vi "Main.vi"(8 "error in (no error)":T1) -> (0 "error out":T1)   [LabVIEW 2019, in "HW Control.lvlib"]
doc: "Confgures and operates mmWave insturment.\nTakes tx data and produces rx data"
uses:
  HW Control.lvlib
  module data.ctl
  SubVIs/mmWave instrument_class/mmWave instrument.lvclass
  SubVIs/Timing_class/Timing.lvclass
  Intertarget communication/UE_slave_class/UE_slave.lvclass
  Intertarget communication/Status + response + data cluster.ctl
  <vilib>/event_ctls.llb/usereventprio.ctl
  SubVIs/mmWave instrument_class/Instrument mode.ctl
  SubVIs/Shared/CMD Configure RF.ctl
  mmw_command_lib/src_LabVIEW/mmW_commands/commands/configure_rf.ctl
  SubVIs/Shared/CMD Configure trigger.ctl
  FPGA/SubVIs/Utility/FPGA driver trigger source.ctl
  FPGA/SubVIs/Utility/FPGA driver trigger destination.ctl
  SubVIs/Low-level/TypeDefs/TX trigger config.ctl
  SubVIs/Shared/CMD SetFS.ctl
  SubVIs/Shared/CMD Enable.ctl
  SubVIs/Shared/CMD Start.ctl
  SubVIs/mmWave HW Control/HW custom error.ctl
  SubVIs/Shared/CMD Trigger burst.ctl
  SubVIs/mmWave instrument_class/BurstMode.ctl
  SubVIs/IQBurst_memo_class/IQBurst_memo.lvclass
  C:/Barkhausen mmWave radar/Development/modules/mmw_instrument/src_LabVIEW/Host/SubVIs/mmWave data_class/mmWave data.lvclass
  5bf6cc24-2521-4779-a80f-885c0f377251.vi
  6b8a8956-422c-4712-ba84-b3f6b6fa3076.vi
  cc201456-c6b0-4b1b-a6be-4740aef1e4bc.vi
  d80f0b82-403c-4990-a471-3ef8a1654657.vi
  00066108-5967-43ca-95ae-979ba40a526a.vi
  dd2405c6-cd62-4e0d-85ef-7dac0ed472a1.vi
  39e6701a-dc6a-46a4-ab36-30c5359b2d1b.vi
  9bb7bbee-87a9-4279-9159-38fc56038457.vi
  5d9b41d4-afd7-4f36-a909-48ea6e6084fe.vi
  c62d52e6-4296-4856-a5ed-4f8c0908956e.vi
  5d74ec58-d27a-4030-a0b1-2ab9eda5ed47.vi
  04c4d11f-ea94-45d4-9853-bbcd34ad9d24.vi
  03bbd1a8-d73e-4344-8b1d-11c8de24bdb2.vi
  b8e4441c-5df3-4338-bc39-36b1f38d4699.vi
  39a1d11b-c092-41e2-b849-1242f73b0438.vi
  25709526-e8ac-4911-9c95-dbb1750b9ebd.vi
  0d6dd9cf-0a41-4f7f-9007-575a6cdc04d9.vi
  c6908804-639b-480e-8665-cc71bcbfa22b.vi
  f746113e-c9c3-4718-88dd-bf493a6a5370.vi
  31d5450a-1eaa-4569-b864-abab59b6c8f0.vi
  0cf5399d-4f5c-45f4-9da5-b5ff7f003509.vi
  ffcc4e67-c424-41ae-a3a8-51a0e91b4a98.vi
  4f1527e8-8d13-40e8-9887-532582f60c4c.vi
  48a184bb-bc8e-4bef-accd-5d588c8dfd0c.vi
  281b50d0-36cb-43e3-a457-c2e31bbdf17e.vi
  6b8a8956-422c-4712-ba84-b3f6b6fa3076.vi/d0b8099d-9a67-487c-8619-7aec39155471.vi
  6b8a8956-422c-4712-ba84-b3f6b6fa3076.vi/4860adc8-6589-4533-9f85-4b2f2f37bc9c.vi
  <vilib>/Utility/High Resolution Relative Seconds.vi
  00066108-5967-43ca-95ae-979ba40a526a.vi/b21b0c59-31bf-4d41-a314-fcb12202764f.vi
  00066108-5967-43ca-95ae-979ba40a526a.vi/59aae4f2-523e-4201-a515-759cc9f383bb.vi
  9bb7bbee-87a9-4279-9159-38fc56038457.vi/ee473946-ddb2-4ec3-8c70-25ef1014e137.vi
  9bb7bbee-87a9-4279-9159-38fc56038457.vi/b9ef59a3-996d-41eb-8d73-01ad8261f39e.vi
  5d9b41d4-afd7-4f36-a909-48ea6e6084fe.vi/0198eef5-db64-4605-ab12-3a788667f18b.vi
  5d9b41d4-afd7-4f36-a909-48ea6e6084fe.vi/f3eba246-8368-4cb8-a50b-49fa0b258f31.vi
  c62d52e6-4296-4856-a5ed-4f8c0908956e.vi/b2fe2695-0bc7-407f-97cd-20d9374a95f4.vi
  c62d52e6-4296-4856-a5ed-4f8c0908956e.vi/e0a517d9-0214-4515-8cec-b207ba4c4c0e.vi
  5d74ec58-d27a-4030-a0b1-2ab9eda5ed47.vi/5a33c0d7-36a7-40b4-9b83-6d2230f6ca4f.vi
  5d74ec58-d27a-4030-a0b1-2ab9eda5ed47.vi/955e3d06-b885-4e3c-85b1-b793e0d77f43.vi
  04c4d11f-ea94-45d4-9853-bbcd34ad9d24.vi/622e0601-9f83-48d3-8254-9b6c5c72482e.vi
  04c4d11f-ea94-45d4-9853-bbcd34ad9d24.vi/4782b8fe-f5f5-46a3-8689-b75fcbd153d5.vi
  03bbd1a8-d73e-4344-8b1d-11c8de24bdb2.vi/af184250-e209-477c-8d9f-d9d37ba09fbc.vi
  03bbd1a8-d73e-4344-8b1d-11c8de24bdb2.vi/336334d0-afb7-43ed-8f90-156a38e6ec86.vi
  25709526-e8ac-4911-9c95-dbb1750b9ebd.vi/ce79f8f7-6f86-47e2-830d-b0a909de7e40.vi
  25709526-e8ac-4911-9c95-dbb1750b9ebd.vi/12f0f21d-a4f0-4ad2-89d4-91e03973e4f6.vi
  0cf5399d-4f5c-45f4-9da5-b5ff7f003509.vi/1adb11cf-635f-40ae-95a1-5f7e8c26521f.vi
  0cf5399d-4f5c-45f4-9da5-b5ff7f003509.vi/b263f872-2439-4497-9f75-8855c3fb30bf.vi
  48a184bb-bc8e-4bef-accd-5d588c8dfd0c.vi/0905219e-2f5e-4d98-acf9-48d7f689f462.vi
  48a184bb-bc8e-4bef-accd-5d588c8dfd0c.vi/bcc9b3b8-3631-40a1-b7b9-ffbaff264bb1.vi
  SubVIs/NISync_class/NISync.lvclass
  C:/Barkhausen mmWave radar/Development/modules/mmw_instrument/src_LabVIEW/Host/SubVIs/Timing_class/Timing.lvclass
  SubVIs/simSync_class/simSync.lvclass
  SubVIs/niMmWave_Transceiver_class/niMmWave_Transceiver.lvclass
  C:/Barkhausen mmWave radar/Development/modules/mmw_instrument/src_LabVIEW/Host/SubVIs/mmWave instrument_class/mmWave instrument.lvclass
  SubVIs/niMmWave_Reciever_class/niMmWave_Reciever.lvclass
  SubVIs/sim_MmW_class/sim_MmW.lvclass
  SubVIs/Shared/Comm GV.vi
  SubVIs/Shared/System GV.vi
  HW GV.vi
  <vilib>/addons/_JKI.lib/Serialization/JSON/Library/Unflatten From JSON String.vi
  Log/Log GV.vi
  SubVIs/mmWave data_class/mmWave data.lvclass
  Intertarget communication/CommandResponse communication.lvlib
  SubVIs/Shared/Shared.lvlib
  FPGA/SubVIs/Utility/FPGA Utility.lvlib
  Data Managment/DataManagment.lvlib
  SubVIs/mmWave HW Control/mmWave HW Control.lvlib
  Log/Log.lvlib
  mmw_command_lib/src_LabVIEW/mmW_commands/mmW_commands.lvlib
panel:
  out "fetch 2":dbl format="%#_6p"
  # "HW Control Main"
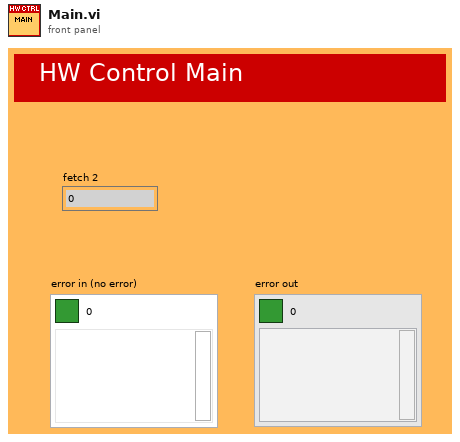
[diagram p1: front panel]
types:
  T1 = cluster{"Boolean Round":bool, "code":i32, "source":string}
  T2 = typedef "CommandResponse communication.lvlib/Status + response + data cluster.ctl" = cluster{"message":string, "response":string, "data":variant}
  T3 = typedef "HW Control.lvlib/module data.ctl" = cluster{"mmWave":refnum<class "mmWave instrument.lvclass">, "timing":refnum<class "Timing.lvclass">, "UE resp":refnum<class "UE_slave.lvclass">}
  T4 = typedef "mmWave instrument.lvclass/Instrument mode.ctl" = enum16{"RF", "IF", "BB"}
  T5 = typedef "usereventprio.ctl" = enum32{"high priority", "normal priority"}
  T6 = typedef "Shared.lvlib/CMD Configure RF.ctl" = cluster{"port":string, "fc":dbl, "gain":dbl}
  T7 = typedef "Shared.lvlib/CMD Configure trigger.ctl" = cluster{"port":string, "delay":dbl, "Trigger source":T8, "Trigger export":T9, "PXI src":i32, "PXI trigger destination":i32}
  T8 = typedef "FPGA Utility.lvlib/FPGA driver trigger source.ctl" = enum16{"Use Tclk", "PXI_Trig", "Aurora RX trig"}
  T9 = typedef "FPGA Utility.lvlib/FPGA driver trigger destination.ctl" = enum16{"None", "Source trig", "Synced trig", "Delayed sync"}
  T10 = typedef "Shared.lvlib/CMD SetFS.ctl" = cluster{"port":string, "fs":dbl}
  T11 = typedef "Shared.lvlib/CMD Enable.ctl" = cluster{"Enable":bool}
  T12 = typedef "Shared.lvlib/CMD Start.ctl" = cluster{"Bursts":string[], "Acquisition duration":dbl}
  T13 = typedef "Shared.lvlib/CMD Trigger burst.ctl" = cluster{"Burst name":string, "Burst mode":T14}
  T14 = typedef "mmWave instrument.lvclass/BurstMode.ctl" = enum16{"burst", "continuous"}
  T15 = typedef "mmW_commands.lvlib/configure_rf.ctl" = cluster{"port":enum16{"rx", "tx"}, "fc":dbl, "gain":dbl, "datatype":string}
  T16 = typedef "TX trigger config.ctl" = cluster{"delay":dbl, "trig source":T8, "PXI src":i32, "export":T9, "PXI dest":i32}
  T17 = cluster{"frequency offset (Hz)":dbl[], "response":cdb[]}
  T18 = typedef "mmWave HW Control.lvlib/HW custom error.ctl" = u16
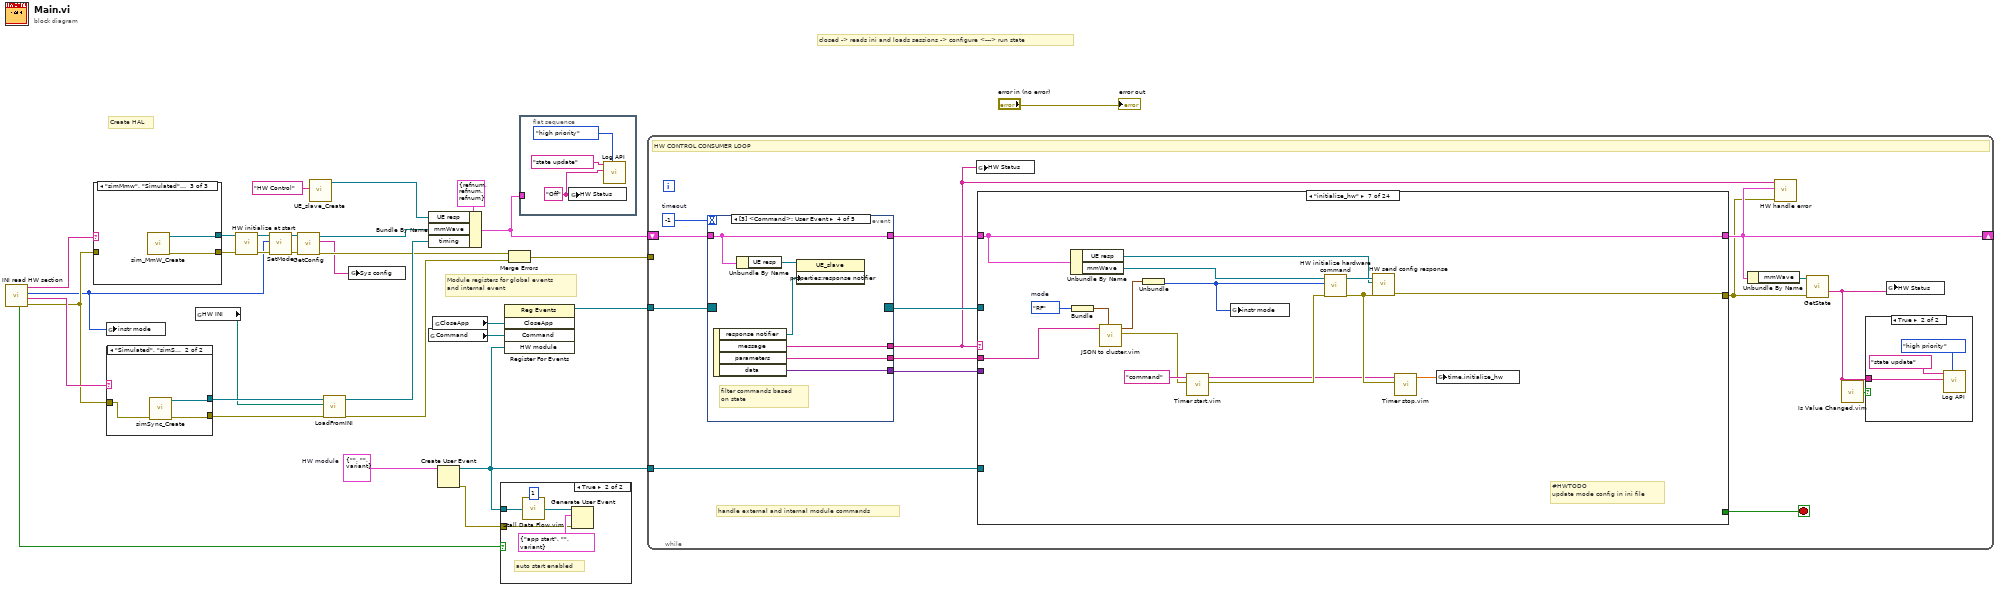
[diagram p0: block diagram]
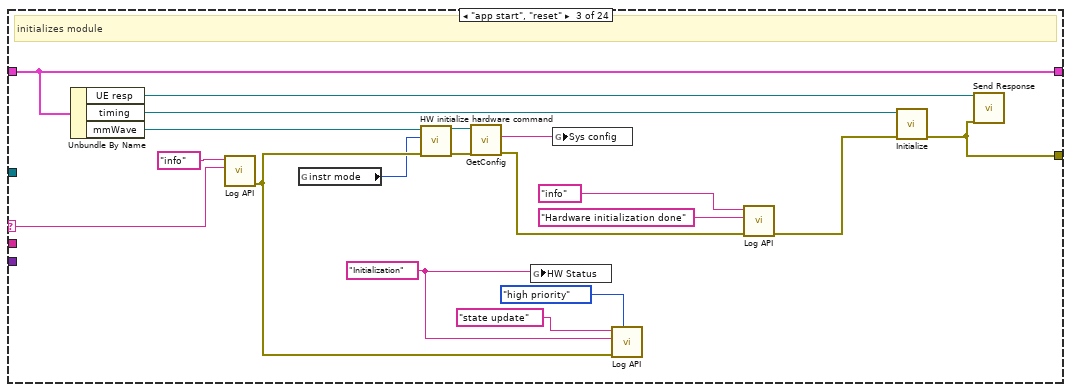
[diagram p6: hidden frame]
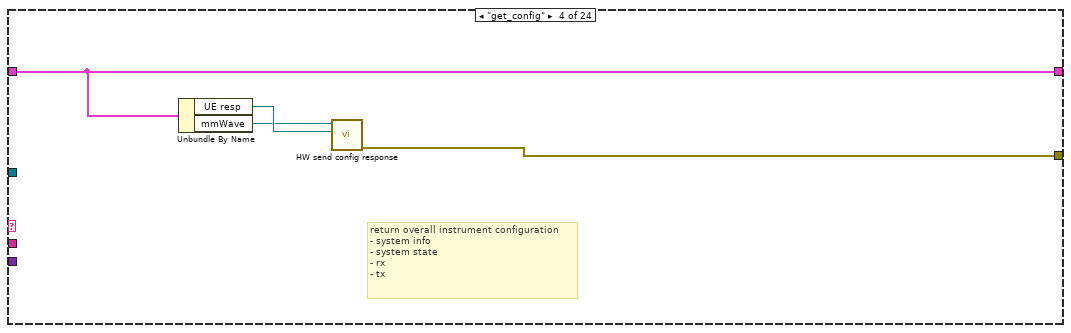
[diagram p7: hidden frame]
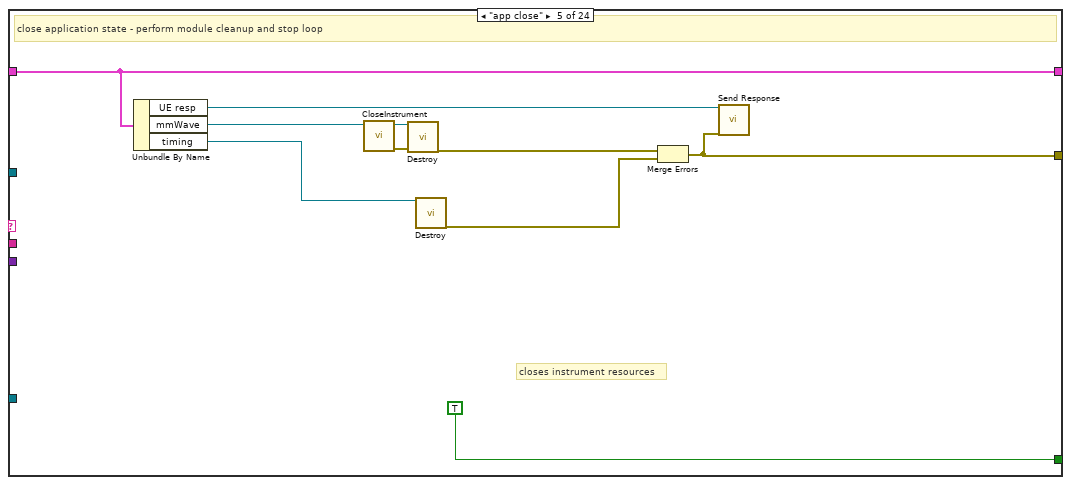
[diagram p8: hidden frame]
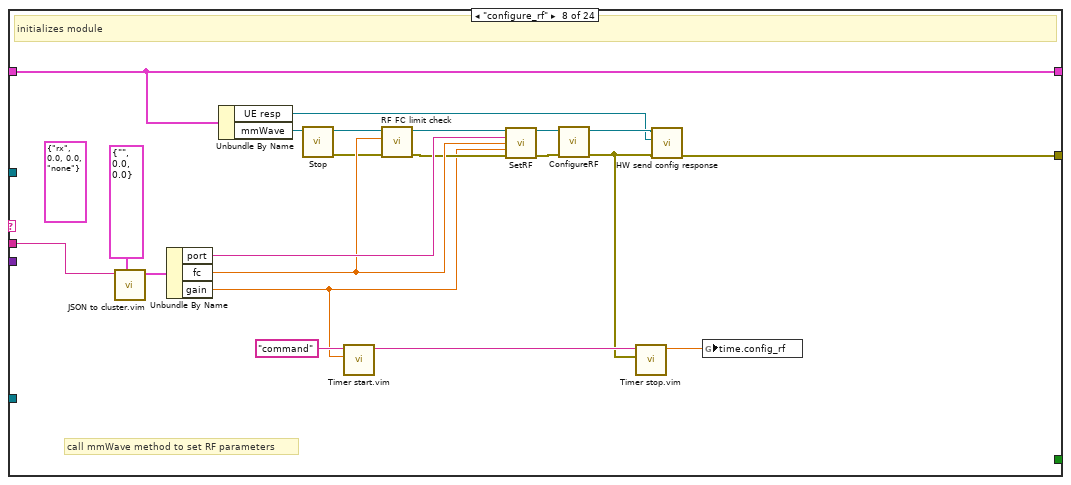
[diagram p10: hidden frame]
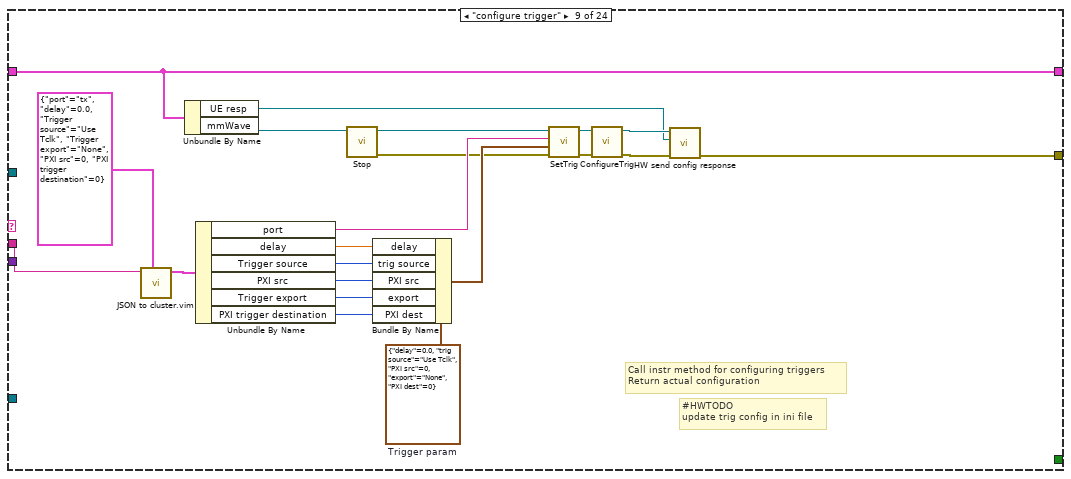
[diagram p11: hidden frame]
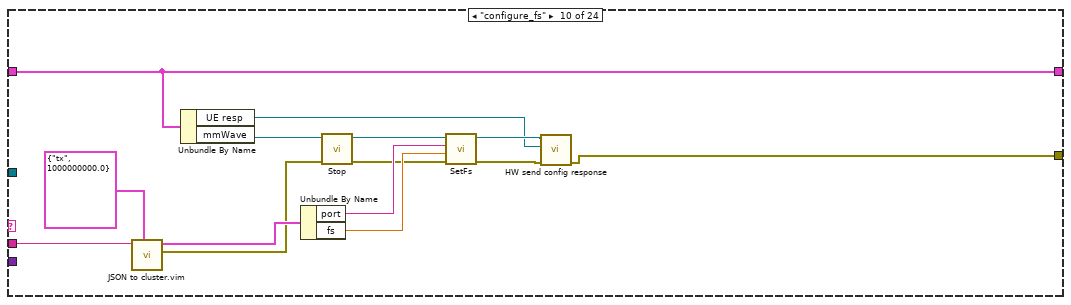
[diagram p12: hidden frame]
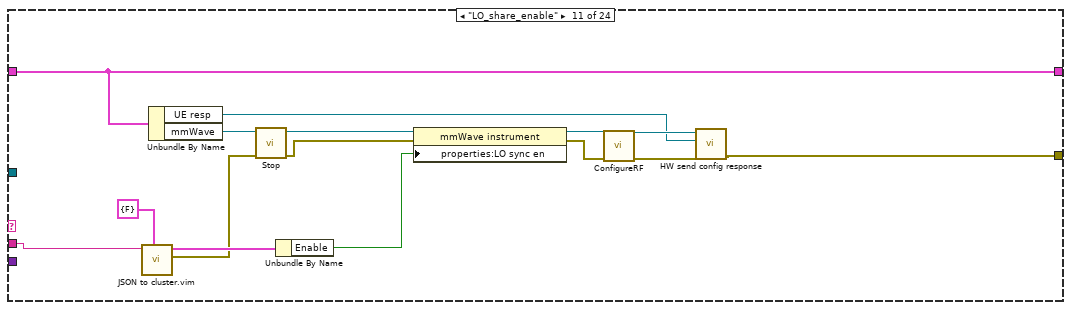
[diagram p13: hidden frame]
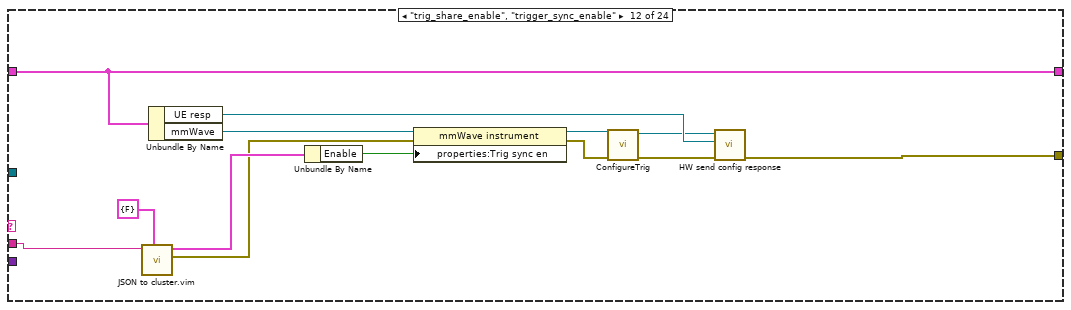
[diagram p14: hidden frame]
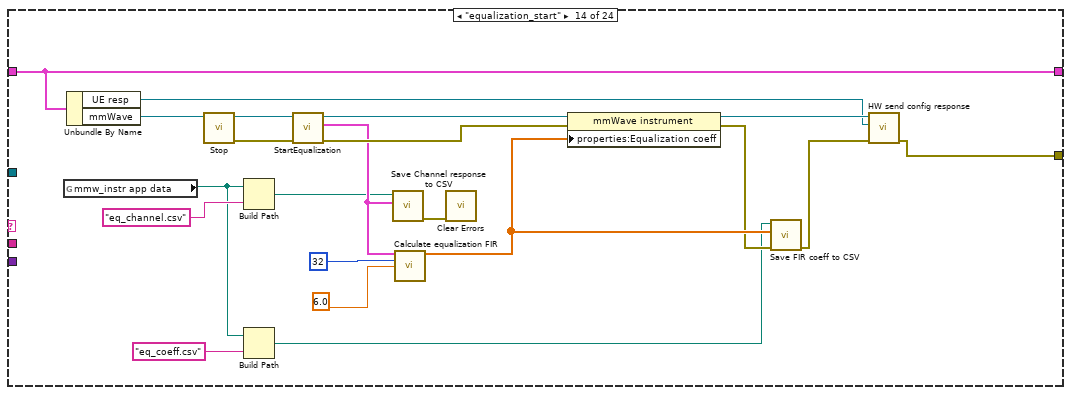
[diagram p16: hidden frame]
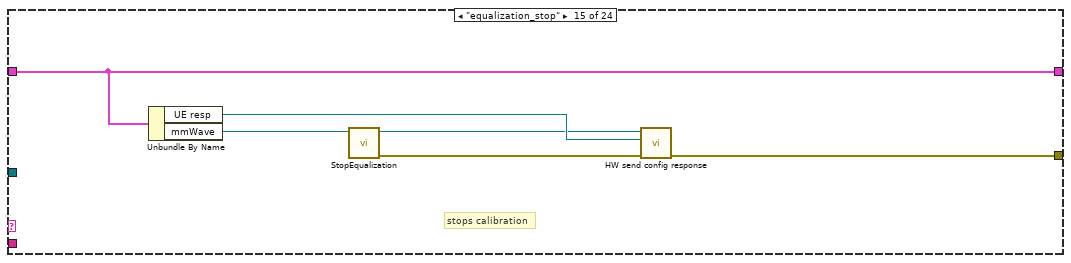
[diagram p17: hidden frame]
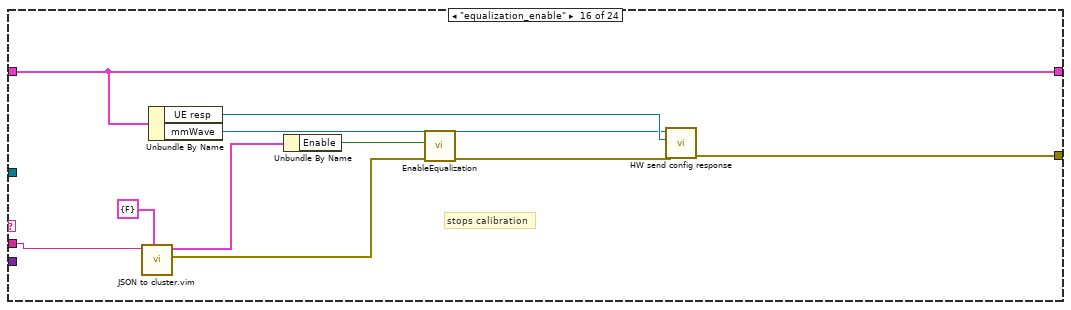
[diagram p18: hidden frame]
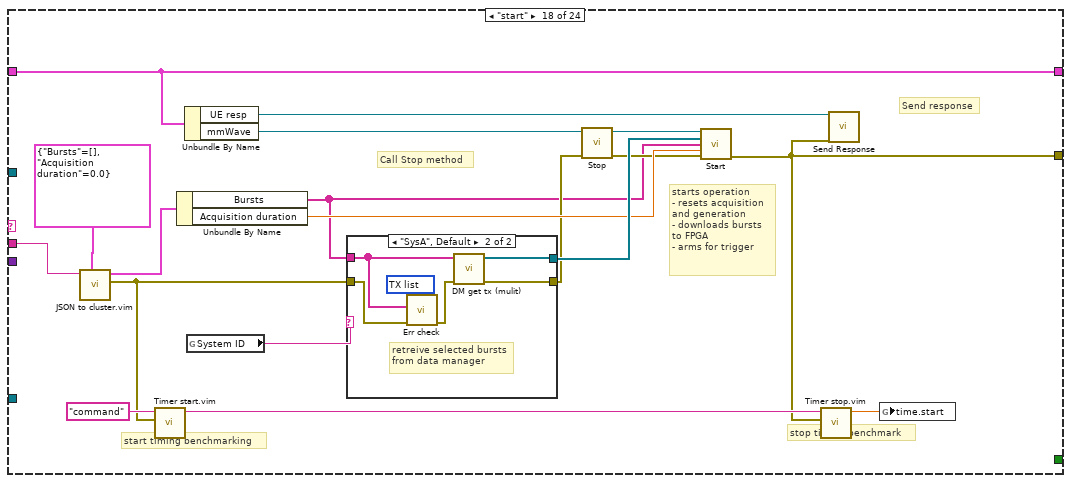
[diagram p20: hidden frame]
diagram:
  w29 = T2 {"message"="", "response"="", "data"=variant}  # HW module
  # "Create HAL"
  # "closed -> reads ini and loads sessions -> configure <---> run state"
  # "Module registers for global events\nand internal event"
  n1 = call "INI read HW section.vi"() -> ("error out"=w23:T1, "timing_class"=w24:string, "instr_mode"=w3:T4, "instr_class"=w25:string, "auto_init"=w6:bool)  [unwired: 7 in]
  n2 = case shown="\"simMmw\", \"Simulated\", Default" w25 {
    tunnel: w23 -> [w34 w37 _]
    tunnel: [w33 w36 w38] -> w11
    tunnel: [w32 w35 w39] -> w12
    frame "niMmWave_Transceiver_class" {
      # "niMmWave\nTransciever"
      n3 = call "niMmWave_Transceiver_Create.vi"("error in (no error)"=w34) -> ("error out"=w33:errorcluster, "reference out"=w32:refnum<class "niMmWave_Transceiver.lvclass">)  [unwired: 9 in]
    }
    frame "niMmWave_Reciever_class" {
      # "niMmWave\nReciever"
      n4 = call "niMmWave_Reciever_Create.vi"("error in (no error)"=w37) -> ("error out"=w36:errorcluster, "reference out"=w35:refnum<class "niMmWave_Reciever.lvclass">)  [unwired: 9 in]
    }
    frame "simMmw", "Simulated", Default {
      n5 = call "sim_MmW_Create.vi"() -> ("error out"=w38:errorcluster, "reference out"=w39:refnum<class "sim_MmW.lvclass">)  [unwired: 10 in]
    }
  }
  n6 = global write "System GV.vi" "instr mode"(w3) -> ()
  n7 = case shown="\"Simulated\", \"simSync\", Default" w24 {
    tunnel: w23 -> [_ w42]
    tunnel: [w40 w43] -> w20
    tunnel: [w41 w44] -> w22
    frame "NISync" {
      # "NISync"
      n8 = call "NISync_Create.vi"() -> ("error out"=w40:errorcluster, "reference out"=w41:refnum<class "NISync.lvclass">)  [unwired: 10 in]
    }
    frame "Simulated", "simSync", Default {
      n9 = call "simSync_Create.vi"("error in (no error)"=w42) -> ("error out"=w43:errorcluster, "reference out"=w44:refnum<class "simSync.lvclass">)  [unwired: 9 in]
    }
  }
  n10 = global read "System GV.vi" "HW INI"() -> (w21:path)
  n11 = call "HW initialize at start.vi"("error in (no error)"=w11, "mmWave instr in"=w12) -> ("error out"=w4:errorcluster, "mmW instr out"=w5:refnum<class "mmWave instrument.lvclass">)  [unwired: 8 in]
  n12 = call-dynamic "SetMode.vi"("error in (no error)"=w4, "instr mode"=w3, "reference in"=w5) -> ("error out"=w1:errorcluster, "reference out"=w2:refnum<class "mmWave instrument.lvclass">)  [unwired: 7 in]
  n13 = call-dynamic "GetConfig.vi"("error in (no error)"=w1, "reference in"=w2) -> ("error out"=w9:errorcluster, "String"=w8:string, "reference out"=w10:refnum<class "mmWave instrument.lvclass">)  [unwired: 7 in]
  n14 = call "UE_slave_Create.vi"("ID"="HW Control") -> ("reference out"=w15:refnum<class "UE_slave.lvclass">)  [unwired: 9 in, 1 out]
  n15 = call-dynamic "LoadFromINI.vi"("error in (no error)"=w20, "Path Control"=w21, "reference in"=w22) -> ("error out"=w17:errorcluster, "reference out"=w19:refnum<class "Timing.lvclass">)  [unwired: 7 in]
  n16 = global write "System GV.vi" "Sys config"(w8) -> ()
  n17 = Bundle By Name(cluster=T3 {"mmWave"=refnum, "timing"=refnum, "UE resp"=refnum} ("module loopdata"), "UE resp"=w15, "mmWave"=w10, "timing"=w19) -> (w13:T3)
  n18 = global read "Comm GV.vi" "Command"() -> (w27:refnum<user-event>)
  n19 = global read "Comm GV.vi" "CloseApp"() -> (w28:refnum<user-event>)
  n20 = Create User Event(user event datatype=w29) -> (user event=w30:refnum<user-event>, error out=w7:errorcluster)  [unwired: 1 in]
  n21 = case shown="True" w6 {
    tunnel: w30 -> [_ w49]
    tunnel: w7 -> [_ w45]
    frame False {
    }
    frame True {
      # "auto start enabled"
      n22 = call "Stall Data Flow.vim"("value in"=w49, "milliseconds to wait"=u32 1) -> ("value out"=w48:refnum<user-event>)  [unwired: 1 out]
      n23 = Generate User Event(user event=w48, event data cluster=T2 {"message"="app start", "response"="", "data"=variant} ("internal command"), error in=w45) -> ()  [unwired: 1 in, 2 out]
    }
  }
  n24 = register-events(w28, w27, w30) -> (reference out=w31:refnum<event-registration>)  [unwired: 2 in, 1 out]
  n25 = Merge Errors(w9, w17) -> (w18:errorcluster)
  n26 = flat-sequence {
    tunnel: w13 -> [_]
    frame #0 {
      w50 = "Off" ("HW Status")
      n27 = global write "HW GV.vi" "HW Status"(w50) -> ()
      n28 = call "Log API.vi"("priority (normal)"=usereventprio."high priority", "data"=w50, "message"="state update") -> ()  [unwired: 8 in, 1 out]
    }
  }
  n29 = while {
    tunnel: w31 -> [w67]
    tunnel: w30 -> [w65]
    shift-right: [w60] -> _
    shift-left: w13 -> [w57]
    tunnel: w18 -> [_]
    stop <- w66 stop-if-true
    w63 = -1  # timeout
    # "handle external and internal module commands"
    # "HW CONTROL CONSUMER LOOP"
    n30 = event shown="[3] <Command>: User Event" {
      selector: w67 -> [_ _ _ _ _]
      dyn-events: [_ _ _ _ _] -> w62
      timeout: w63 -> [_ _ _ _ _]
      tunnel: ["" ("message") "app close" "close" w370 w374] -> w61
      tunnel: [_ _ _ w371 w373] -> w64
      tunnel: w57 -> [w359 w361 w363 w369 w372]
      tunnel: [w359 w361 w363 w369 w372] -> w56
      tunnel: [_ _ _ w366 _] -> w55
      event Timeout {
        n31 = event-data() -> ()  [unwired: 1 in, 1 out]
      }
      event User Event {
        n32 = event-data() -> ()  [unwired: 1 in, 1 out]
      }
      event Panel Close? {
        n33 = event-data() -> ()  [unwired: 1 in, 1 out]
        n34 = event-data("Discard?"=TRUE) -> ()  [unwired: 1 in, 1 out]
      }
      event User Event {
        # "filter commands based\non state"
        n35 = event-data() -> ("response notifier"=w367:refnum<notifier>, "message"=w370:string, "parameters"=w371:string, "data"=w366:variant)  [unwired: 1 in]
        n36 = Unbundle By Name(w369) -> ("UE resp"=w368:refnum<class "UE_slave.lvclass">)
        n37 = property class="UE_slave"(reference=w368, "properties:response notifier"=w367) -> ()  [unwired: 1 in, 2 out]
      }
      event User Event {
        n38 = event-data() -> ("message"=w374:string, "response"=w373:string)  [unwired: 1 in]
      }
    }
    n39 = global write "HW GV.vi" "HW Status"(w61) -> ()
    n40 = case shown="\"initialize_hw\"" w61 {
      selector: w61 -> [_ _ w85 _ _ _ _ _ _ _ _ _ _ _ _ _ _ _ _ _ _ _ _ _]
      tunnel: [_ _ _ _ TRUE _ _ _ _ _ _ _ _ _ _ _ _ _ _ _ _ _ _ _] -> w66
      tunnel: w65 -> [_ _ _ _ _ _ _ _ _ _ _ _ _ _ _ _ _ _ _ _ _ _ _ _]
      tunnel: w56 -> [w71 w72 w91 w95 w104 w106 w122 w143 w164 w178 w193 w206 w207 w228 w234 w245 w246 w264 w293 w309 w326 w330 w357 w358]
      tunnel: [w71 w72 w91 w95 w104 w106 w122 w143 w164 w178 w193 w206 w207 w228 w234 w245 w246 w264 w293 w309 w326 w330 w357 w358] -> w60
      tunnel: w64 -> [_ _ _ _ _ _ w120 w141 w163 w177 w191 w203 _ _ _ w243 _ w262 w290 _ w323 _ w353 _]
      tunnel: [_ _ w87 w92 w96 _ w113 w128 w144 w165 w181 w194 _ w208 w229 w235 _ w247 w279 w301 w317 w327 w334 _] -> w58
      tunnel: w62 -> [_ _ _ _ _ _ _ _ _ _ _ _ _ _ _ _ _ _ _ _ _ _ _ _]
      tunnel: w55 -> [_ _ _ _ _ _ _ _ _ _ _ _ _ _ _ _ _ _ _ _ _ _ w356 _]
      frame Default {
      }
      frame "----APP CONTROL----" {
      }
      frame "app start", "reset" {
        w81 = "Initialization" ("HW Status")
        # "initializes module"
        n41 = Unbundle By Name(w91) -> ("UE resp"=w90:refnum<class "UE_slave.lvclass">, "timing"=w89:refnum<class "Timing.lvclass">, "mmWave"=w88:refnum<class "mmWave instrument.lvclass">)
        n42 = call "Log API.vi"("data"=w85, "message"="info") -> ("error out"=w78:T1)  [unwired: 9 in]
        n43 = global read "System GV.vi" "instr mode"() -> (w77:T4)
        n44 = call "HW initialize hardware command.vi"("error in (no error)"=w78, "mode"=w77, "mmWave instrument in"=w88) -> ("error out"=w76:errorcluster, "mmWave instrument out"=w75:refnum<class "mmWave instrument.lvclass">)  [unwired: 7 in]
        n45 = call-dynamic "GetConfig.vi"("error in (no error)"=w76, "reference in"=w75) -> ("error out"=w74:errorcluster, "String"=w73:string)  [unwired: 7 in, 1 out]
        n46 = global write "HW GV.vi" "HW Status"(w81) -> ()
        n47 = global write "System GV.vi" "Sys config"(w73) -> ()
        n48 = call "Log API.vi"("priority (normal)"=usereventprio."high priority", "error in (no error)"=w78, "data"=w81, "message"="state update") -> ()  [unwired: 7 in, 1 out]
        n49 = call "Log API.vi"("error in (no error)"=w74, "data"="Hardware initialization done", "message"="info") -> ("error out"=w84:T1)  [unwired: 8 in]
        n50 = call-dynamic "Initialize.vi"("error in (no error)"=w84, "reference in"=w89) -> ("error out"=w87:errorcluster)  [unwired: 8 in, 1 out]
        n51 = call-dynamic "Send Response.vi"("reference in"=w90, "error in (no error)"=w87) -> ()  [unwired: 16 in, 2 out]
      }
      frame "get_config" {
        # "return overall instrument configuration\n- system info\n- system state\n- rx\n- tx"
        n52 = Unbundle By Name(w95) -> ("UE resp"=w94:refnum<class "UE_slave.lvclass">, "mmWave"=w93:refnum<class "mmWave instrument.lvclass">)
        n53 = call "HW send config response.vi"("UE resp"=w94, "mmWave instrument in"=w93) -> ("error out"=w92:errorcluster)  [unwired: 9 in]
      }
      frame "app close" {
        # "closes instrument resources"
        # "close application state - perform module cleanup and stop loop"
        n54 = Unbundle By Name(w104) -> ("UE resp"=w97:refnum<class "UE_slave.lvclass">, "mmWave"=w102:refnum<class "mmWave instrument.lvclass">, "timing"=w99:refnum<class "Timing.lvclass">)
        n55 = call-dynamic "CloseInstrument.vi"("reference in"=w102) -> ("error out"=w101:errorcluster, "reference out"=w103:refnum<class "mmWave instrument.lvclass">)  [unwired: 9 in]
        n56 = call-dynamic "Destroy.vi"("reference in"=w103, "error in (no error)"=w101) -> ("error out"=w100:errorcluster)  [unwired: 16 in, 1 out]
        n57 = call-dynamic "Destroy.vi"("reference in"=w99) -> ("error out"=w98:errorcluster)  [unwired: 17 in, 1 out]
        n58 = Merge Errors(w100, w98) -> (w96:errorcluster)
        n59 = call-dynamic "Send Response.vi"("reference in"=w97, "error in (no error)"=w96) -> ()  [unwired: 16 in, 2 out]
      }
      frame "----CONFIGURE----" {
        # "Configure commands placeholder"
      }
      frame "initialize_hw" {
        w121 = Instrument_mode."RF"  # mode
        # "#HWTODO\nupdate mode config in ini file"
        n60 = Unbundle By Name(w122) -> ("UE resp"=w114:refnum<class "UE_slave.lvclass">, "mmWave"=w117:refnum<class "mmWave instrument.lvclass">)
        n61 = Bundle("mode"=w121) -> (w119:cluster{"mode":T4})  [unwired: 1 in]
        n62 = call "JSON to cluster.vim"("data"=w119, "JSON in"=w120) -> ("error out"=w111:errorcluster, "data"=w118:cluster{"mode":T4})  [unwired: 7 in, 1 out]
        n63 = Unbundle(w118) -> ("mode"=w116:T4)
        n64 = call "Timer start.vim"("dataflow in"=w111, "timer in (t1)"="command" ("timer name (t1)")) -> ("dataflow out"=w110:errorcluster, "timer out"=w108:string)  [unwired: 8 in]
        n65 = global write "System GV.vi" "instr mode"(w116) -> ()
        n66 = call "HW initialize hardware command.vi"("error in (no error)"=w110, "mode"=w116, "mmWave instrument in"=w117) -> ("error out"=w109:errorcluster, "mmWave instrument out"=w115:refnum<class "mmWave instrument.lvclass">)  [unwired: 7 in]
        n67 = call "HW send config response.vi"("error in (no error)"=w109, "UE resp"=w114, "mmWave instrument in"=w115) -> ("error out"=w113:errorcluster)  [unwired: 8 in]
        n68 = call "Timer stop.vim"("dataflow in"=w109, "timer name (t1)"=w108) -> ("final time"=w107:dbl)  [unwired: 8 in, 1 out]
        n69 = global write "Log GV.vi" "time.initialize_hw"(w107) -> ()
      }
      frame "configure_rf" {
        (unwired) T15 {"port"=enum."rx", "fc"=0.0, "gain"=0.0, "datatype"="none"} ("Cluster")
        # "call mmWave method to set RF parameters"
        # "initializes module"
        n70 = call "JSON to cluster.vim"("data"=T6 {"port"="", "fc"=0.0, "gain"=0.0}, "JSON in"=w141) -> ("data"=w139:T6)  [unwired: 7 in, 2 out]
        n71 = Unbundle By Name(w139) -> ("port"=w137:string, "fc"=w133:dbl, "gain"=w124:dbl)
        n72 = Unbundle By Name(w143) -> ("UE resp"=w129:refnum<class "UE_slave.lvclass">, "mmWave"=w142:refnum<class "mmWave instrument.lvclass">)
        n73 = call-dynamic "Stop.vi"("reference in"=w142) -> ("error out"=w132:errorcluster, "reference out"=w135:refnum<class "mmWave instrument.lvclass">)  [unwired: 9 in]
        n74 = call "Timer start.vim"("dataflow in"=w124, "timer in (t1)"="command" ("timer name (t1)")) -> ("timer out"=w126:string)  [unwired: 8 in, 1 out]
        n75 = call-dynamic "RF FC limit check.vi"("error in (no error)"=w132, "RF Fc"=w133, "reference in"=w135) -> ("error out"=w131:errorcluster, "reference out"=w134:refnum<class "mmWave instrument.lvclass">)  [unwired: 7 in]
        n76 = call-dynamic "SetRF.vi"("reference in"=w134, "Port"=w137, "Frequency"=w133, "Gain"=w124, "error in (no error)"=w131) -> ("reference out"=w138:refnum<class "mmWave instrument.lvclass">, "error out"=w136:errorcluster)  [unwired: 9 in]
        n77 = call-dynamic "ConfigureRF.vi"("error in (no error)"=w136, "reference in"=w138) -> ("error out"=w123:errorcluster, "reference out"=w130:refnum<class "mmWave instrument.lvclass">)  [unwired: 8 in]
        n78 = call "Timer stop.vim"("dataflow in"=w123, "timer name (t1)"=w126) -> ("final time"=w125:dbl)  [unwired: 8 in, 1 out]
        n79 = call "HW send config response.vi"("error in (no error)"=w123, "UE resp"=w129, "mmWave instrument in"=w130) -> ("error out"=w128:errorcluster)  [unwired: 8 in]
        n80 = global write "Log GV.vi" "time.config_rf"(w125) -> ()
      }
      frame "configure trigger" {
        w160 = T16 {"delay"=0.0, "trig source"=enum."Use Tclk", "PXI src"=0, "export"=enum."None", "PXI dest"=0}  # Trigger param
        # "#HWTODO\nupdate trig config in ini file"
        # "Call instr method for configuring triggers\nReturn actual configuration"
        n81 = call "JSON to cluster.vim"("data"=T7 {"port"="tx", "delay"=0.0, "Trigger source"=enum."Use Tclk", "Trigger export"=enum."None", "PXI src"=0, "PXI trigger destination"=0}, "JSON in"=w163) -> ("data"=w161:T7)  [unwired: 7 in, 2 out]
        n82 = Unbundle By Name(w164) -> ("UE resp"=w146:refnum<class "UE_slave.lvclass">, "mmWave"=w150:refnum<class "mmWave instrument.lvclass">)
        n83 = Unbundle By Name(w161) -> ("port"=w153:string, "delay"=w159:dbl, "Trigger source"=w158:T8, "PXI src"=w157:i32, "Trigger export"=w156:T9, "PXI trigger destination"=w155:i32)
        n84 = call-dynamic "Stop.vi"("reference in"=w150) -> ("error out"=w148:errorcluster, "reference out"=w149:refnum<class "mmWave instrument.lvclass">)  [unwired: 9 in]
        n85 = Bundle By Name(cluster=w160, "delay"=w159, "trig source"=w158, "PXI src"=w157, "export"=w156, "PXI dest"=w155) -> (w152:T16)
        n86 = call-dynamic "SetTrig.vi"("error in (no error)"=w148, "TX trigger options"=w152, "Port"=w153, "reference in"=w149) -> ("error out"=w151:errorcluster, "reference out"=w154:refnum<class "mmWave instrument.lvclass">)  [unwired: 6 in]
        n87 = call-dynamic "ConfigureTrig.vi"("error in (no error)"=w151, "reference in"=w154) -> ("error out"=w145:errorcluster, "reference out"=w147:refnum<class "mmWave instrument.lvclass">)  [unwired: 8 in]
        n88 = call "HW send config response.vi"("error in (no error)"=w145, "UE resp"=w146, "mmWave instrument in"=w147) -> ("error out"=w144:errorcluster)  [unwired: 8 in]
      }
      frame "configure_fs" {
        n89 = call "JSON to cluster.vim"("data"=T10 {"port"="tx", "fs"=1000000000.0} ("Set fs command"), "JSON in"=w177) -> ("error out"=w170:errorcluster, "data"=w174:T10)  [unwired: 7 in, 1 out]
        n90 = Unbundle By Name(w178) -> ("UE resp"=w166:refnum<class "UE_slave.lvclass">, "mmWave"=w176:refnum<class "mmWave instrument.lvclass">)
        n91 = Unbundle By Name(w174) -> ("port"=w173:string, "fs"=w172:dbl)
        n92 = call-dynamic "Stop.vi"("error in (no error)"=w170, "reference in"=w176) -> ("error out"=w169:errorcluster, "reference out"=w171:refnum<class "mmWave instrument.lvclass">)  [unwired: 8 in]
        n93 = call-dynamic "SetFs.vi"("error in (no error)"=w169, "Fs"=w172, "Port"=w173, "reference in"=w171) -> ("error out"=w168:errorcluster, "reference out"=w167:refnum<class "mmWave instrument.lvclass">)  [unwired: 6 in]
        n94 = call "HW send config response.vi"("error in (no error)"=w168, "UE resp"=w166, "mmWave instrument in"=w167) -> ("error out"=w165:errorcluster)  [unwired: 8 in]
      }
      frame "LO_share_enable" {
        n95 = call "JSON to cluster.vim"("data"=T11 {"Enable"=FALSE} ("Equalization command"), "JSON in"=w191) -> ("error out"=w184:errorcluster, "data"=w190:T11)  [unwired: 7 in, 1 out]
        n96 = Unbundle By Name(w193) -> ("UE resp"=w179:refnum<class "UE_slave.lvclass">, "mmWave"=w188:refnum<class "mmWave instrument.lvclass">)
        n97 = call-dynamic "Stop.vi"("error in (no error)"=w184, "reference in"=w188) -> ("error out"=w183:errorcluster, "reference out"=w185:refnum<class "mmWave instrument.lvclass">)  [unwired: 8 in]
        n98 = Unbundle By Name(w190) -> ("Enable"=w187:bool)
        n99 = property class="mmWave instrument"(reference=w185, error in=w183, "properties:LO sync en"=w187) -> (reference out=w186:refnum<class "mmWave instrument.lvclass">, error out=w192:errorcluster)
        n100 = call-dynamic "ConfigureRF.vi"("error in (no error)"=w192, "reference in"=w186) -> ("error out"=w182:errorcluster, "reference out"=w180:refnum<class "mmWave instrument.lvclass">)  [unwired: 8 in]
        n101 = call "HW send config response.vi"("error in (no error)"=w182, "UE resp"=w179, "mmWave instrument in"=w180) -> ("error out"=w181:errorcluster)  [unwired: 8 in]
      }
      frame "trig_share_enable", "trigger_sync_enable" {
        n102 = call "JSON to cluster.vim"("data"=T11 {"Enable"=FALSE} ("Equalization command"), "JSON in"=w203) -> ("error out"=w201:errorcluster, "data"=w202:T11)  [unwired: 7 in, 1 out]
        n103 = Unbundle By Name(w206) -> ("UE resp"=w205:refnum<class "UE_slave.lvclass">, "mmWave"=w199:refnum<class "mmWave instrument.lvclass">)
        n104 = Unbundle By Name(w202) -> ("Enable"=w198:bool)
        n105 = property class="mmWave instrument"(reference=w199, error in=w201, "properties:Trig sync en"=w198) -> (reference out=w197:refnum<class "mmWave instrument.lvclass">, error out=w204:errorcluster)
        n106 = call-dynamic "ConfigureTrig.vi"("error in (no error)"=w204, "reference in"=w197) -> ("error out"=w195:errorcluster, "reference out"=w196:refnum<class "mmWave instrument.lvclass">)  [unwired: 8 in]
        n107 = call "HW send config response.vi"("error in (no error)"=w195, "UE resp"=w205, "mmWave instrument in"=w196) -> ("error out"=w194:errorcluster)  [unwired: 8 in]
      }
      frame "----EQUALIZATION----" {
      }
      frame "equalization_start" {
        n108 = global read "System GV.vi" "mmw_instr app data"() -> (w213:path)
        n109 = Unbundle By Name(w228) -> ("UE resp"=w210:refnum<class "UE_slave.lvclass">, "mmWave"=w223:refnum<class "mmWave instrument.lvclass">)
        n110 = call-dynamic "Stop.vi"("reference in"=w223) -> ("error out"=w221:errorcluster, "reference out"=w222:refnum<class "mmWave instrument.lvclass">)  [unwired: 9 in]
        n111 = Build Path(base path=w213, name or relative path="eq_channel.csv") -> (appended path=w215:path)
        n112 = Build Path(base path=w213, name or relative path="eq_coeff.csv") -> (appended path=w212:path)
        n113 = call-dynamic "StartEqualization.vi"("error in (no error)"=w221, "reference in"=w222) -> ("error out"=w224:errorcluster, "channel"=w218:T17, "reference out"=w225:refnum<class "mmWave instrument.lvclass">)  [unwired: 7 in]
        n114 = call "Save Channel response to CSV.vi"("channel"=w218, "Path"=w215) -> ("error out"=w217:T1)  [unwired: 9 in]
        n115 = call "Calculate equalization FIR.vi"("channel"=w218, "FIR taps"=32, "Max FIR gain"=6.0) -> ("EQ FIR coeff"=w220:cdb[])  [unwired: 10 in, 2 out]
        n116 = call <vilib>:"Clear Errors.vi"("error in (no error)"=w217) -> ()  [unwired: 5 in, 2 out]
        n117 = property class="mmWave instrument"(reference=w225, error in=w224, "properties:Equalization coeff"=w220) -> (reference out=w211:refnum<class "mmWave instrument.lvclass">, error out=w219:errorcluster)
        n118 = call "Save FIR coeff to CSV.vi"("error in (no error)"=w219, "EQ FIR coeff"=w220, "Path"=w212) -> ("error out"=w209:T1)  [unwired: 8 in]
        n119 = call "HW send config response.vi"("error in (no error)"=w209, "UE resp"=w210, "mmWave instrument in"=w211) -> ("error out"=w208:errorcluster)  [unwired: 8 in]
      }
      frame "equalization_stop" {
        # "stops calibration"
        n120 = Unbundle By Name(w234) -> ("UE resp"=w232:refnum<class "UE_slave.lvclass">, "mmWave"=w233:refnum<class "mmWave instrument.lvclass">)
        n121 = call-dynamic "StopEqualization.vi"("reference in"=w233) -> ("error out"=w230:errorcluster, "reference out"=w231:refnum<class "mmWave instrument.lvclass">)  [unwired: 9 in]
        n122 = call "HW send config response.vi"("error in (no error)"=w230, "UE resp"=w232, "mmWave instrument in"=w231) -> ("error out"=w229:errorcluster)  [unwired: 8 in]
      }
      frame "equalization_enable" {
        # "stops calibration"
        n123 = call "JSON to cluster.vim"("data"=T11 {"Enable"=FALSE} ("Equalization command"), "JSON in"=w243) -> ("error out"=w240:errorcluster, "data"=w242:T11)  [unwired: 7 in, 1 out]
        n124 = Unbundle By Name(w245) -> ("UE resp"=w238:refnum<class "UE_slave.lvclass">, "mmWave"=w244:refnum<class "mmWave instrument.lvclass">)
        n125 = Unbundle By Name(w242) -> ("Enable"=w241:bool)
        n126 = call-dynamic "EnableEqualization.vi"("error in (no error)"=w240, "Enable/Disable"=w241, "reference in"=w244) -> ("error out"=w236:errorcluster, "reference out"=w237:refnum<class "mmWave instrument.lvclass">)  [unwired: 7 in]
        n127 = call "HW send config response.vi"("error in (no error)"=w236, "UE resp"=w238, "mmWave instrument in"=w237) -> ("error out"=w235:errorcluster)  [unwired: 8 in]
      }
      frame "----RUN----" {
      }
      frame "start" {
        # "Send response"
        # "Call Stop method"
        # "stop timing benchmark"
        # "start timing benchmarking"
        # "starts operation\n- resets acquisition \nand generation\n- downloads bursts\nto FPGA\n- arms for trigger"
        n128 = call "JSON to cluster.vim"("data"=T12 {"Bursts"=[], "Acquisition duration"=0.0} ("Start command"), "JSON in"=w262) -> ("error out"=w248:errorcluster, "data"=w261:T12)  [unwired: 7 in, 1 out]
        n129 = call "Timer start.vim"("dataflow in"=w248, "timer in (t1)"="command" ("timer name (t1)")) -> ("timer out"=w250:string)  [unwired: 8 in, 1 out]
        n130 = Unbundle By Name(w261) -> ("Bursts"=w252:string[], "Acquisition duration"=w259:dbl)
        n131 = Unbundle By Name(w264) -> ("UE resp"=w258:refnum<class "UE_slave.lvclass">, "mmWave"=w256:refnum<class "mmWave instrument.lvclass">)
        n132 = global read "System GV.vi" "System ID"() -> (w257:string)
        n133 = case shown="\"SysA\", Default" w257 {
          tunnel: w252 -> [_ w266]
          tunnel: [_ w271] -> w263
          tunnel: [w265 w270] -> w254
          tunnel: w248 -> [w265 w268]
          frame "SysB" {
            # "do not retrieve\nbursts for sysB"
          }
          frame "SysA", Default {
            w269 = T18 10000 items=["TX list"=10000, "TX length"=10001, "RX length"=10002] ("HW custom err")
            # "retreive selected bursts\nfrom data manager"
            n134 = call "Err check.vi"("error in"=w268, "Variant Control"=w266, "HW custom err"=w269) -> ("error out"=w267:errorcluster)  [unwired: 8 in]
            n135 = call "DM get tx (mulit).vi"("error in (no error)"=w267, "tx bursts"=w266) -> ("error out"=w270:errorcluster, "1D Array"=w271:refnum<class "mmWave data.lvclass">[])  [unwired: 8 in]
          }
        }
        n136 = call-dynamic "Stop.vi"("error in (no error)"=w254, "reference in"=w256) -> ("error out"=w253:errorcluster, "reference out"=w255:refnum<class "mmWave instrument.lvclass">)  [unwired: 8 in]
        n137 = call-dynamic "Start.vi"("reference in"=w255, "TX bursts"=w263, "sequence"=w252, "RX acq length"=w259, "error in (no error)"=w253) -> ("error out"=w247:errorcluster)  [unwired: 9 in, 1 out]
        n138 = call "Timer stop.vim"("dataflow in"=w247, "timer name (t1)"=w250) -> ("final time"=w249:dbl)  [unwired: 8 in, 1 out]
        n139 = call-dynamic "Send Response.vi"("reference in"=w258, "error in (no error)"=w247) -> ()  [unwired: 16 in, 2 out]
        n140 = global write "Log GV.vi" "time.start"(w249) -> ()
      }
      frame "trigger_burst" {
        # "- Trigger burst generation\n- Fetch RX data\n- Send data to data managment module\n- send command response"
        n141 = global read "System GV.vi" "System ID"() -> (w288:string)
        n142 = call "JSON to cluster.vim"("data"=T13 {"Burst name"="", "Burst mode"=enum."burst"} ("Trigger burst command"), "JSON in"=w290) -> ("error out"=w282:errorcluster, "data"=w283:T13)  [unwired: 7 in, 1 out]
        n143 = Concatenate Strings(w288, " rx" ("group")) -> (w286:string)
        n144 = Unbundle By Name(w283) -> ("Burst mode"=w289:T14)  [unwired: 1 out]
        n145 = Unbundle By Name(w293) -> ("UE resp"=w284:refnum<class "UE_slave.lvclass">, "mmWave"=w292:refnum<class "mmWave instrument.lvclass">)
        n146 = call-dynamic "GenerateBurst.vi"("error in (no error)"=w282, "Burst mode"=w289, "reference in"=w292) -> ("error out"=w276:errorcluster, "reference out"=w285:refnum<class "mmWave instrument.lvclass">)  [unwired: 7 in]
        n147 = call "Timer start.vim"("dataflow in"=w276, "timer in (t1)"="fetch" ("timer name (t1)")) -> ("dataflow out"=w275:errorcluster)  [unwired: 8 in, 1 out]
        n148 = call-dynamic "FetchRX.vi"("error in (no error)"=w275, "reference in"=w285) -> ("error out"=w281:errorcluster, "RX burst data"=w274:refnum<class "mmWave data.lvclass">)  [unwired: 7 in, 1 out]
        n149 = call "Timer stop.vim"("dataflow in"=w274, "timer name (t1)"="fetch") -> ("final time"=→"fetch 2":dbl)  [unwired: 8 in, 1 out]
        n150 = call-dynamic "Send Response.vi"("reference in"=w284, "data"=w274, "error in (no error)"=w281) -> ("error out"=w278:errorcluster)  [unwired: 15 in, 1 out]
        n151 = call "Send data.vi"("error in (no error)"=w281, "group"=w286, "Data"=w274) -> ("error out"=w280:T1)  [unwired: 8 in]
        n152 = Merge Errors(w278, w280) -> (w279:errorcluster)
      }
      frame "fetch" {
        # "- Fetch RX data\n- Send data to data managment module\n- send command response"
        n153 = Unbundle By Name(w309) -> ("UE resp"=w305:refnum<class "UE_slave.lvclass">, "mmWave"=w299:refnum<class "mmWave instrument.lvclass">)
        n154 = call "Timer start.vim"("dataflow in"=w299, "timer in (t1)"="fetch" ("timer name (t1)")) -> ("dataflow out"=w298:refnum<class "mmWave instrument.lvclass">)  [unwired: 8 in, 1 out]
        n155 = global read "System GV.vi" "System ID"() -> (w308:string)
        n156 = Concatenate Strings(w308, " rx" ("group")) -> (w306:string)
        n157 = call-dynamic "FetchRX.vi"("reference in"=w298) -> ("error out"=w303:errorcluster, "RX burst data"=w304:refnum<class "mmWave data.lvclass">)  [unwired: 8 in, 1 out]
        n158 = call-dynamic "Send Response.vi"("reference in"=w305, "data"=w304, "error in (no error)"=w303) -> ("reference out"=w296:refnum<class "UE_slave.lvclass">, "error out"=w300:errorcluster)  [unwired: 15 in]
        n159 = call "Send data.vi"("error in (no error)"=w303, "group"=w306, "Data"=w304) -> ("error out"=w302:T1)  [unwired: 8 in]
        n160 = call "Timer stop.vim"("dataflow in"=w296, "timer name (t1)"="fetch") -> ("final time"=w294:dbl)  [unwired: 8 in, 1 out]
        n161 = Merge Errors(w300, w302) -> (w301:errorcluster)
        n162 = global write "Log GV.vi" "time.fetch"(w294) -> ()
      }
      frame "send_trigger" {
        # "- Trigger burst generation\n- Fetch RX data\n- Send data to data managment module\n- send command response"
        n163 = global read "System GV.vi" "System ID"() -> (w321:string)
        n164 = call "JSON to cluster.vim"("data"=T13 {"Burst name"="", "Burst mode"=enum."burst"} ("Trigger burst command"), "JSON in"=w323) -> ("error out"=w312:errorcluster, "data"=w318:T13)  [unwired: 7 in, 1 out]
        n165 = Concatenate Strings(w321, " rx" ("group")) -> ()  [unwired: 1 out]
        n166 = Unbundle By Name(w318) -> ("Burst mode"=w322:T14)
        n167 = Unbundle By Name(w326) -> ("UE resp"=w319:refnum<class "UE_slave.lvclass">, "mmWave"=w325:refnum<class "mmWave instrument.lvclass">)
        n168 = call "Timer start.vim"("dataflow in"=w312, "timer in (t1)"="command" ("timer name (t1)")) -> ("dataflow out"=w311:errorcluster, "timer out"=w314:string)  [unwired: 8 in]
        n169 = call-dynamic "GenerateBurst.vi"("error in (no error)"=w311, "Burst mode"=w322, "reference in"=w325) -> ("error out"=w310:errorcluster)  [unwired: 7 in, 1 out]
        n170 = call "Timer stop.vim"("dataflow in"=w310, "timer name (t1)"=w314) -> ("final time"=w313:dbl)  [unwired: 8 in, 1 out]
        n171 = call-dynamic "Send Response.vi"("reference in"=w319, "error in (no error)"=w310) -> ("error out"=w316:errorcluster)  [unwired: 16 in, 1 out]
        n172 = global write "Log GV.vi" "time.send_trig"(w313) -> ()
        n173 = Merge Errors(w316, w310) -> (w317:errorcluster)
      }
      frame "stop" {
        # "stops tx generation\nand rx fetching"
        n174 = Unbundle By Name(w330) -> ("UE resp"=w328:refnum<class "UE_slave.lvclass">, "mmWave"=w329:refnum<class "mmWave instrument.lvclass">)
        n175 = call-dynamic "Stop.vi"("reference in"=w329) -> ("error out"=w327:errorcluster)  [unwired: 9 in, 1 out]
        n176 = call-dynamic "Send Response.vi"("reference in"=w328, "error in (no error)"=w327) -> ()  [unwired: 16 in, 2 out]
      }
      frame "transcieve" {
        n177 = call "JSON to cluster.vim"("data"=T12 {"Bursts"=[], "Acquisition duration"=0.0} ("Start command"), "JSON in"=w353) -> ("error out"=w344:errorcluster, "data"=w355:T12)  [unwired: 7 in, 1 out]
        n178 = Unbundle By Name(w357) -> ("UE resp"=w345:refnum<class "UE_slave.lvclass">, "mmWave"=w343:refnum<class "mmWave instrument.lvclass">)
        n179 = Unbundle By Name(w355) -> ("Bursts"=w331:string[], "Acquisition duration"=w352:dbl)
        n180 = Variant To Data(error in=w344, type=refnum<class "IQBurst_memo.lvclass"> refnum ("reference out"), Variant=w356) -> (data=w338:refnum<class "IQBurst_memo.lvclass">, error out=w333:errorcluster)
        n181 = call-dynamic "Stop.vi"("reference in"=w343) -> ("reference out"=w342:refnum<class "mmWave instrument.lvclass">)  [unwired: 9 in, 1 out]
        n182 = call-dynamic "GetObjectStatus.vi"("reference in"=w338, "simple info (F)"=TRUE, "error in (no error)"=w333) -> ("reference out"=w336:refnum<class "IQBurst_memo.lvclass">, "error out"=w332:errorcluster)  [unwired: 5 in, 10 out]
        n183 = call "Send data.vi"("error in (no error)"=w333, "group"="tx", "Data"=w338) -> ()  [unwired: 8 in, 1 out]
        n184 = Build Array(w336) -> (w351:refnum<class "IQBurst_memo.lvclass">[])
        n185 = call-dynamic "Start.vi"("reference in"=w342, "TX bursts"=w351, "sequence"=w331, "RX acq length"=w352, "error in (no error)"=w332) -> ("reference out"=w348:refnum<class "mmWave instrument.lvclass">, "error out"=w347:errorcluster)  [unwired: 9 in]
        n186 = call-dynamic "GenerateBurst.vi"("error in (no error)"=w347, "reference in"=w348) -> ("error out"=w349:errorcluster, "reference out"=w350:refnum<class "mmWave instrument.lvclass">)  [unwired: 8 in]
        n187 = call-dynamic "FetchRX.vi"("error in (no error)"=w349, "reference in"=w350) -> ("error out"=w339:errorcluster, "RX burst data"=w337:refnum<class "mmWave data.lvclass">)  [unwired: 7 in, 1 out]
        n188 = call-dynamic "Send Response.vi"("reference in"=w345, "data"=w337, "error in (no error)"=w339) -> ()  [unwired: 15 in, 2 out]
        n189 = call "Send data.vi"("error in (no error)"=w339, "group"="rx", "Data"=w337) -> ("error out"=w334:T1)  [unwired: 8 in]
      }
      frame "----CLEANUP----" {
      }
    }
    n190 = Unbundle By Name(w60) -> ("mmWave"=w59:refnum<class "mmWave instrument.lvclass">)
    n191 = call "HW handle error.vi"("error in (no error)"=w58, "module loopdata"=w60, "command"=w61) -> ()  [unwired: 9 in]
    n192 = call-dynamic "GetState.vi"("reference in"=w59, "error in (no error)"=w58) -> ("state (str)"=w53:string)  [unwired: 9 in, 4 out]
    n193 = call "Is Value Changed.vim"("value"=w53) -> ("changed or first call?"=w54:bool)
    n194 = case shown="True" w54 {
      tunnel: w53 -> [_ w69]
      frame False {
      }
      frame True {
        n195 = call "Log API.vi"("priority (normal)"=usereventprio."high priority", "data"=w69, "message"="state update") -> ()  [unwired: 8 in, 1 out]
      }
    }
    n196 = global write "HW GV.vi" "HW Status"(w53) -> ()
  }
  "error out" <- "error in (no error)"
